vi "Get Slave Configuration File from User.vi"(8 "error in":errorcluster) -> (0 "error out":errorcluster, 3 "Test Config":T3={"Chopper RPM"=140, "IR Power"=5, "Conc Tolerance"=0.0, "Gas Stable Time"=0, "A-D Settle"=0, "Samples"=0, "Filter Time"=0, "Gas Mixtures"=[], "Filter Sequences"=[], "Functional Test"={"Mic Test ON ADC Max"=0.0, "Mic Test ON ADC Min"=0.0, "Mic Test OFF ADC Max"=0.0, "Mic Test OFF ADC Min"=0.0, "Mic Test IC ADC Max"=0.0, "Mic Test IC ADC Min"=0.0, "IR Emitter ON ADC Max"=0.0, "IR Emitter ON ADC Min"=0.0, "IR Emitter OFF ADC Max"=0.0, "IR Emitter OFF ADC Min"=0.0}, "Initial Flow Rate"=0.0, "Max Flow Rate"=0.0} {"Gas Mixtures"."ADC Gains" items=["0"=0, "3"=3, "4"=4, "5"=5, "6"=6, "7"=7]; "Conc Tolerance" min=0.0 max=100.0 step=1.0; "IR Power" min=2 max=5 step=1; "Chopper RPM" min=140 max=1000 step=1}, 5 "selected path":path, 7 "Master Config":T1 {"Conc Tolerance" min=0.0 max=100.0 step=1.0})   [LabVIEW 2015]
uses:
  Controls/Test Config.ctl
  Controls/Gas Mixture.ctl
  CAN Communication/PAS/Typedefs/ADC Gains.ctl
  Controls/Filter Sequence.ctl
  Controls/Functional Test.ctl
  Controls/Master Config.ctl
  Controls/Gas Info.ctl
  CAN Communication/PAS/PAS.lvclass
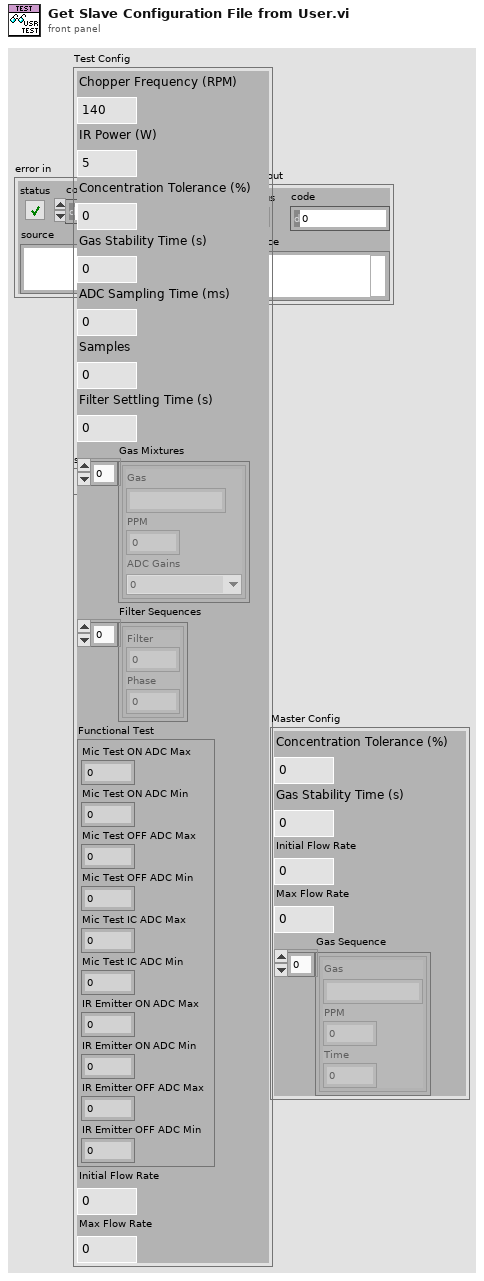
[diagram p1: front panel]
types:
  T1 = typedef "Master Config.ctl" = cluster{"Conc Tolerance":dbl, "Gas Stable Time":u16, "Initial Flow Rate":sgl, "Max Flow Rate":sgl, "Gas Sequence":T2[]}
  T2 = typedef "Gas Info.ctl" = cluster{"Gas":string, "PPM":dbl, "Time":u32}
  T3 = typedef "Test Config.ctl" = cluster{"Chopper RPM":u16, "IR Power":u8, "Conc Tolerance":dbl, "Gas Stable Time":u16, "A-D Settle":u16, "Samples":u16, "Filter Time":u16, "Gas Mixtures":T4[], "Filter Sequences":T6[], "Functional Test":T7, "Initial Flow Rate":sgl, "Max Flow Rate":sgl}
  T4 = typedef "Gas Mixture.ctl" = cluster{"Gas":string, "PPM":dbl, "ADC Gains":T5}
  T5 = typedef "PAS.lvclass/ADC Gains.ctl" = u16
  T6 = typedef "Filter Sequence.ctl" = cluster{"Filter":u8, "Phase":dbl}
  T7 = typedef "Functional Test.ctl" = cluster{"Mic Test ON ADC Max":dbl, "Mic Test ON ADC Min":dbl, "Mic Test OFF ADC Max":dbl, "Mic Test OFF ADC Min":dbl, "Mic Test IC ADC Max":dbl, "Mic Test IC ADC Min":dbl, "IR Emitter ON ADC Max":dbl, "IR Emitter ON ADC Min":dbl, "IR Emitter OFF ADC Max":dbl, "IR Emitter OFF ADC Min":dbl}
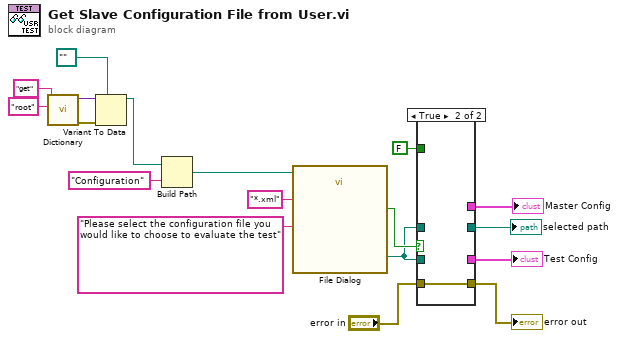
[diagram p0: block diagram]
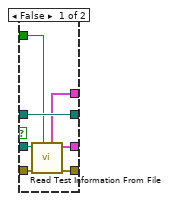
[diagram p2: hidden frame]
diagram:
  n1 = call "Dictionary.vi"("Key"="root", "Command"="get") -> ("error out"=w4:errorcluster, "Value Out"=w3:variant)  [unwired: 8 in]
  n2 = Variant To Data(error in=w4, type=path "" ("appended path"), Variant=w3) -> (data=w1:path)  [unwired: 1 out]
  n3 = Build Path(base path=w1, name or relative path="Configuration") -> (appended path=w17:path)
  n4 = call "File Dialog"("start path"=w17, "prompt"="Please select the configuration file you would like to choose to evaluate the test", "pattern (all files)"="*.xml") -> ("selected path"=w11:path, "cancelled"=w13:bool)  [unwired: 9 in, 2 out]
  n5 = case shown="True" w13 {
    tunnel: "error in" -> [w25 w26]
    tunnel: w11 -> [w24 _]
    tunnel: [w23 _] -> w9
    tunnel: [w22 w26] -> w14
    tunnel: [w21 _] -> w10
    tunnel: w11 -> [w21 _]
    tunnel: [w20 _] -> w8
    tunnel: FALSE ("Master?") -> [w19 _]
    frame False {
      n6 = call "Read Test Information From File.vi"("Master?"=w19, "error in"=w25, "file (use dialog)"=w24) -> ("error out"=w22:errorcluster, "Test Config"=w23:T3, "Master Config"=w20:T1)  [unwired: 6 in]
    }
    frame True {
    }
  }
  "error out" <- w14
  "selected path" <- w10
  "Test Config" <- w9
  "Master Config" <- w8
